vi "8点端铆试验判定.vi"(7 "Result":refnum<vi>, 9 "判定参数":T1, 10 "XY曲线 2":cluster{"X":dbl[], "Y":dbl[]}[](array[cluster]), 11 "XY曲线":cluster{"X":dbl[], "Y":dbl[]}[](array[cluster])) -> (2 "判定项长度":i32, 3 "OK？":bool)   [LabVIEW 2020]
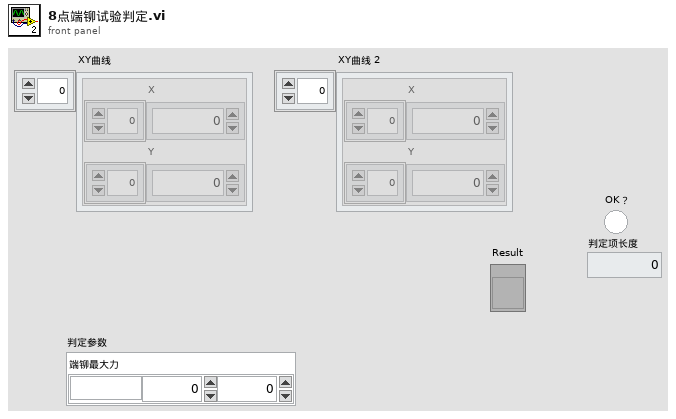
[diagram p1: front panel]
types:
  T1 = cluster{"端铆最大力":cluster{"单位":string, "下限":dbl, "上限":dbl}}
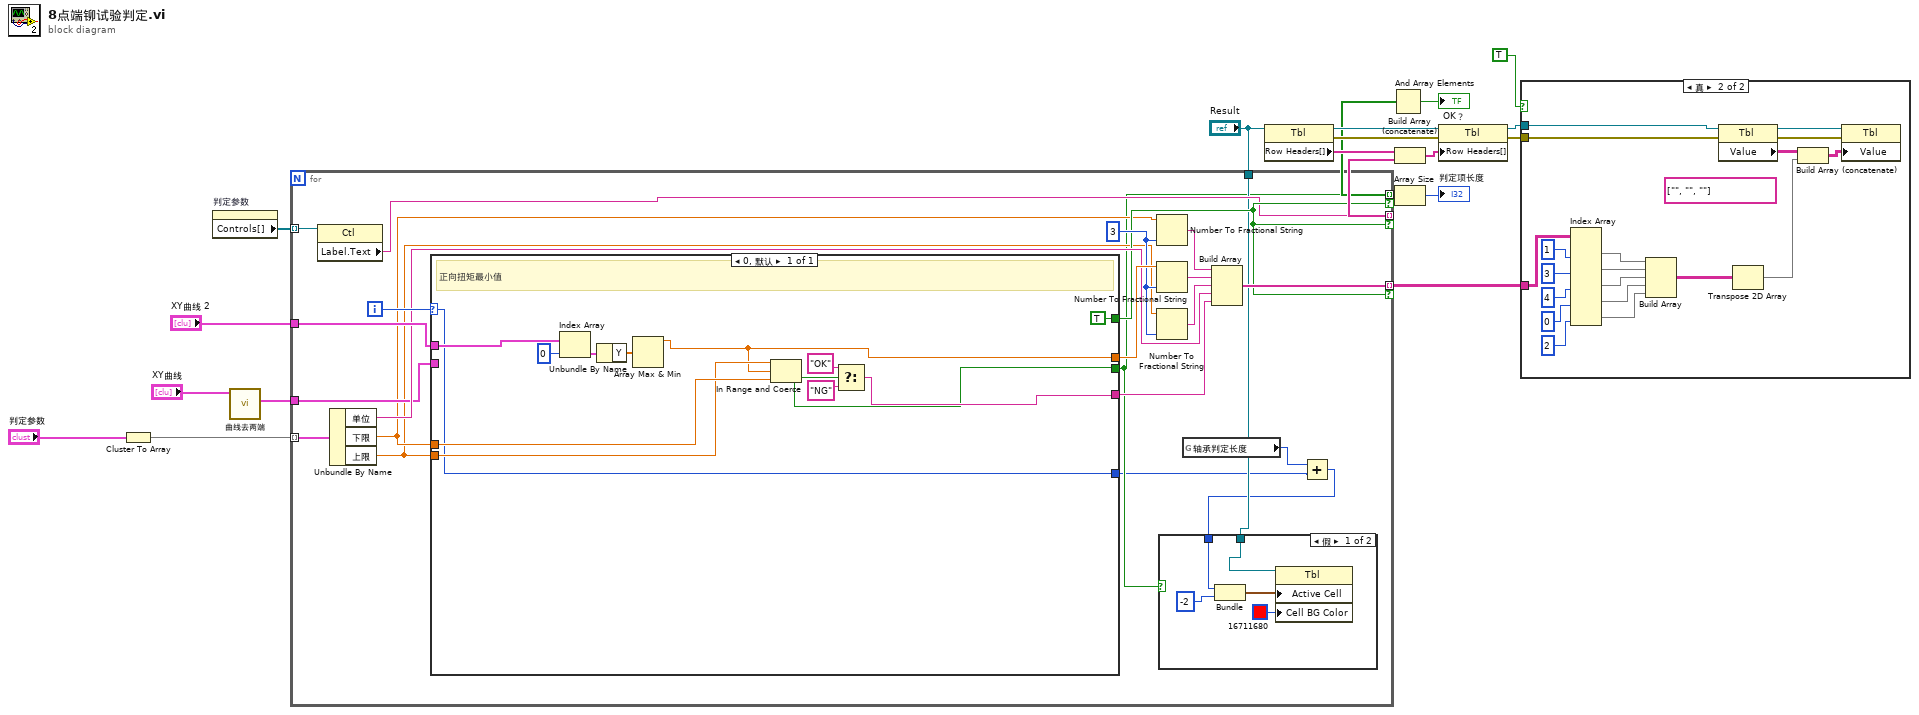
[diagram p0: block diagram]
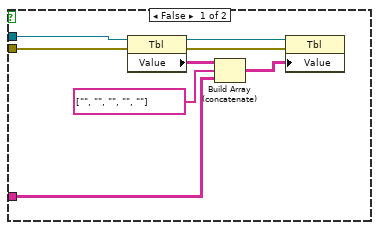
[diagram p2: hidden frame]
diagram:
  n1 = Cluster To Array(cluster="判定参数") -> (array=w19:cluster{"单位":string, "下限":dbl, "上限":dbl}[])
  n2 = property on="判定参数" class="Clust (严格)"() -> ("Controls[]"=w9:refnum<vi>[])  [unwired: 2 in, 2 out]
  n3 = call "曲线去两端.vi"("曲线In"="XY曲线") -> ("启动曲线"=w5:cluster{"X":dbl[], "Y":dbl[]}[])  [unwired: 9 in, 1 out]
  n4 = for {
    tunnel: w19 -> [w41] mode=indexing
    tunnel: w9 -> [w39] mode=indexing
    tunnel: "XY曲线 2" -> [w37]
    tunnel: [w23] -> w7 mode=indexing if=w29
    tunnel: [w30] -> w10 mode=indexing if=w29
    tunnel: [w25] -> w12 mode=indexing if=w29
    tunnel: w5 -> [w28]
    tunnel: "Result" -> [w24]
    i -> [w40]
    w36 = i16 3 ("精度(6)")
    n5 = property class="Ctl"(reference=w39) -> ("Label.Text"=w25:string)  [unwired: 1 in, 2 out]
    n6 = Unbundle By Name(w41) -> ("单位"=w31:string, "下限"=w27:dbl, "上限"=w26:dbl)
    n7 = case shown="0, 默认" w40 {
      selector: w40 -> [w47]
      tunnel: [w48] -> w38
      tunnel: w37 -> [w59]
      tunnel: [w55] -> w32
      tunnel: [w54] -> w23
      tunnel: w27 -> [w53]
      tunnel: w26 -> [w52]
      tunnel: [TRUE] -> w29
      tunnel: w28 -> [_]
      tunnel: [w47] -> w21
      frame 0, Default {
        # "正向扭矩最小值"
        n8 = Index Array(array=w59, index=0 ("索引")) -> (element=w58:cluster{"X":dbl[], "Y":dbl[]})
        n9 = Unbundle By Name(w58) -> ("Y"=w50:dbl[])
        n10 = Array Max & Min(array=w50) -> (max value=w48:dbl)  [unwired: 3 out]
        n11 = In Range and Coerce(upper limit=w52, x=w48, lower limit=w53) -> (In Range?=w54:bool)  [unwired: 1 out]
        n12 = Select(t="OK", s=w54, f="NG") -> (s? t:f=w55:string)
      }
    }
    n13 = Number To Fractional String(number=w27, precision (6)=w36) -> (F-format string=w35:string)  [unwired: 2 in]
    n14 = Number To Fractional String(number=w38, precision (6)=w36) -> (F-format string=w34:string)  [unwired: 2 in]
    n15 = Number To Fractional String(number=w26, precision (6)=w36) -> (F-format string=w33:string)  [unwired: 2 in]
    n16 = global read "判定参数.vi" "轴承判定长度"() -> (w22:i32)
    n17 = Build Array(w35, w34, w33, w31, w32) -> (w30:string[])
    n18 = Add(x=w22, y=w21) -> (x+y=w20:i32)
    n19 = case shown="假" w23 {
      tunnel: w24 -> [w46 _]
      tunnel: w20 -> [w42 _]
      frame False {
        n20 = Bundle(w42, "索引"=-2) -> (w43:cluster{i32, "索引":i32})  [unwired: 1 in]
        n21 = property class="Tbl"(reference=w46, "Active Cell"=w43, "Cell BG Color"=u32 16711680 ("活动单元格:单元格背景色")) -> ()  [unwired: 1 in, 2 out]
      }
      frame True {
      }
    }
  }
  n22 = property class="Tbl"(reference="Result") -> (reference out=w14:refnum<vi>, error out=w17:errorcluster, "Row Headers[]"=w11:string[])  [unwired: 1 in]
  n23 = And Array Elements(Boolean array=w7) -> (logical AND=→"OK？":bool)
  n24 = Build Array (concatenate)(w11, w12) -> (w13:string[])
  n25 = Array Size(array=w7) -> (size(s)=→"判定项长度":i32)
  n26 = property class="Tbl"(reference=w14, error in=w17, "Row Headers[]"=w13) -> (reference out=w15:refnum<vi>, error out=w16:errorcluster)
  n27 = case shown="真" TRUE {
    tunnel: w16 -> [w65 w84]
    tunnel: w15 -> [w62 w81]
    tunnel: w10 -> [w61 w80]
    frame False {
      n28 = property class="Tbl"(reference=w62, error in=w65) -> (reference out=w63:refnum<vi>, error out=w64:errorcluster, "Value"=w66:string[][])
      n29 = Build Array (concatenate)(w66, string[] ["", "", "", "", ""], w61) -> (w67:string[][])
      n30 = property class="Tbl"(reference=w63, error in=w64, "Value"=w67) -> ()  [unwired: 2 out]
    }
    frame True {
      (unwired) string[] ["", "", ""]
      n31 = Index Array(array=w80, index (col) #1=1 ("禁用的索引 (列)"), index (col) #2=3 ("索引 (列)"), index (col) #3=4 ("索引 (列)"), index (col) #4=0 ("索引 (列)"), index (col) #5=2 ("索引 (列)")) -> (element #1=w76:string[], element #2=w75:string[], element #3=w74:string[], element #4=w69:string[], element #5=w68:string[])  [unwired: 5 in]
      n32 = Build Array(w76, w75, w74, w69, w68) -> (w73:string[][])
      n33 = property class="Tbl"(reference=w81, error in=w84) -> (reference out=w82:refnum<vi>, error out=w83:errorcluster, "Value"=w85:string[][])
      n34 = Transpose 2D Array(2D array=w73) -> (transposed array=w72:string[][])
      n35 = Build Array (concatenate)(w85, w72) -> (w86:string[][])
      n36 = property class="Tbl"(reference=w82, error in=w83, "Value"=w86) -> ()  [unwired: 2 out]
    }
  }
